vi "SPI_GetMaxSpeed.vi"(5 "Device":i32, 7 "Bus":i32=1, 8 "error in":errorcluster) -> (0 "error out":errorcluster, 4 "max speed (Hz)":u32)   [LabVIEW 2014]
doc: "Reads the maximum speed for the specified SPI device."
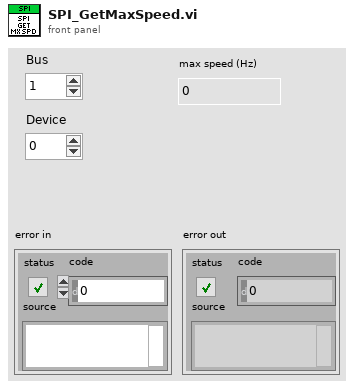
[diagram p1: front panel]
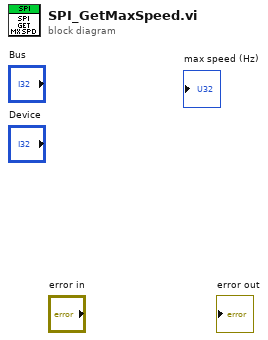
[diagram p0: block diagram]
diagram:
